vi "STFT by Indices.vi"(0 "scaled signal [EU]":dbl[](array[numeric]) format="%.2f", 1 "indices":i32[](array[numeric]), 2 "FFT block size":i32=1024, 5 "sampling frequency [Hz]":dbl=10000.0 format="%.2f", 7 "frequency weighting":T3(ring), 9 "window":T2 items=["Rectangle"=0, "Hanning"=1, "Hamming"=2, "Blackman-Harris"=3, "Exact Blackman"=4, "Blackman"=5, "Flat Top"=6, "4 Term B-Harris "=7, "7 Term B-Harris"=8, "Low Sidelobe"=9, "Blackman Nuttall"=11, "Triangle"=30, "Bartlett-Hanning"=31, "Bohman"=32, "Parzen"=33, "Welch"=34, "Kaiser"=60, "Dolph-Chebyshev"=61, "Gaussian"=62], 11 "channel info":T1={"sensor sensitivity [mV/EU]"=1000.0, "engineering units"=enum."V", "dB reference [EU]"=1.0, "custom label"="EU", "weighting filter"=enum."Linear", "pregain [dB]"=0.0} {"dB reference [EU]" format="%.1e"; "pregain [dB]" format="%.2f"; "sensor sensitivity [mV/EU]" format="%.2f"}, 12 "dB On (T)":bool=TRUE) -> (4 "power spectrum [EU^2 rms]":dbl[][](array[numeric]) format="%.2f", 6 "unit label":string, 8 "f0 and delta f [Hz]":cluster{"f0":dbl, "delta f":dbl} {"delta f" format="%.2f"; "f0" format="%.2f"}, 15 "weighting conflict":bool)   [LabVIEW 2017]
uses:
  <vilib>/Analysis/4window.llb/windowTd.ctl
  <vilib>/Analysis/NI_AALPro.lvlib
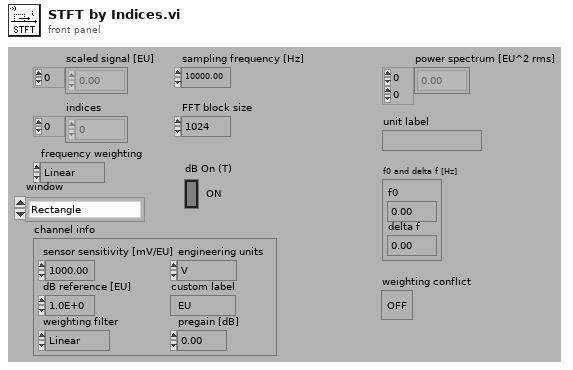
[diagram p1: front panel]
types:
  T1 = cluster{"sensor sensitivity [mV/EU]":dbl, "engineering units":enum16{"custom...", "V", "Pa", "g", "m/s^2", "m/s", "m", "in/s^2", "in/s", "in"}, "dB reference [EU]":dbl, "custom label":string, "weighting filter":enum16{"Linear", "A-weighting", "B-weighting", "C-weighting"}, "pregain [dB]":dbl}
  T2 = typedef "NI_AALPro.lvlib/windowTd.ctl" = u32
  T3 = enum16{"Linear", "A-weighting", "B-weighting", "C-weighting"}
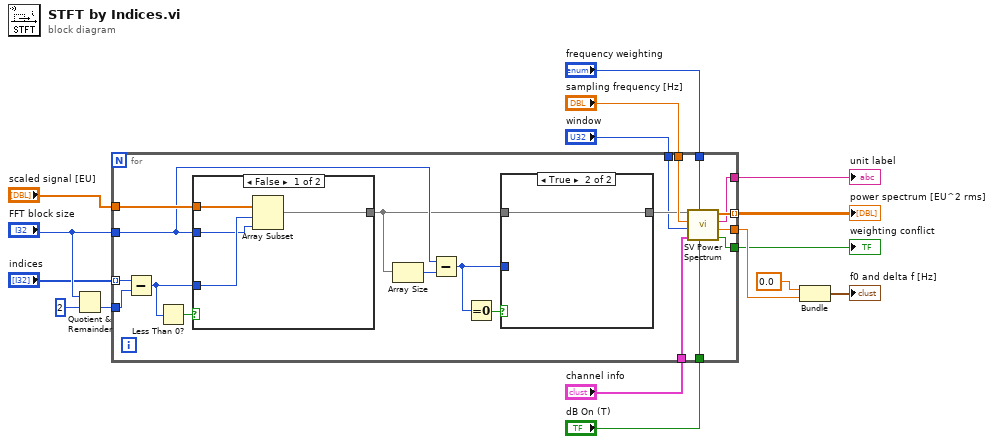
[diagram p0: block diagram]
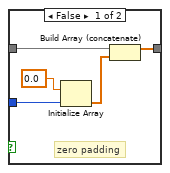
[diagram p2: hidden frame]
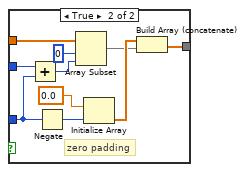
[diagram p3: hidden frame]
diagram:
  n1 = Quotient & Remainder(x="FFT block size", y=2) -> (floor(x/y)=w15:i32)  [unwired: 1 out]
  n2 = for {
    tunnel: w15 -> [w36]
    tunnel: "scaled signal [EU]" -> [w34]
    tunnel: "FFT block size" -> [w33]
    tunnel: "sampling frequency [Hz]" -> [w30]
    tunnel: [w29] -> w14 mode=indexing
    tunnel: [w27] -> w13
    tunnel: "frequency weighting" -> [w23]
    tunnel: "window" -> [w22]
    tunnel: "channel info" -> [w21]
    tunnel: "dB On (T)" -> [w20]
    tunnel: [w19] -> w5
    tunnel: [w18] -> w4
    tunnel: "indices" -> [w17] mode=indexing
    n3 = Subtract(x=w17, y=w36) -> (x-y=w35:i32)
    n4 = Less Than 0?(x=w35) -> (x < 0?=w28:bool)
    n5 = case shown="False" w28 {
      tunnel: w35 -> [w45 w52]
      tunnel: w34 -> [w46 w54]
      tunnel: w33 -> [w44 w50]
      tunnel: [w43 w47] -> w32
      frame False {
        n6 = Array Subset(array=w46, index=w45, length=w44) -> (w43:dbl[])
      }
      frame True {
        # "zero padding"
        n7 = Add(x=w50, y=w52) -> (x+y=w51:i32)
        n8 = Negate(x=w52) -> (-x=w56:i32)
        n9 = Array Subset(array=w54, index=0, length=w51) -> (w48:dbl[])
        n10 = Initialize Array(0.0, w56) -> (w49:dbl[])
        n11 = Build Array (concatenate)(w49, w48) -> (w47:dbl[])
      }
    }
    n12 = Array Size(array=w32) -> (size(s)=w26:i32)
    n13 = Subtract(x=w33, y=w26) -> (x-y=w31:i32)
    n14 = Equal To 0?(x=w31) -> (x = 0?=w25:bool)
    n15 = case shown="True" w25 {
      tunnel: [w37 w42] -> w24
      tunnel: w32 -> [w41 w42]
      tunnel: w31 -> [w39 _]
      frame False {
        # "zero padding"
        n16 = Initialize Array(0.0, w39) -> (w38:dbl[])
        n17 = Build Array (concatenate)(w41, w38) -> (w37:dbl[])
      }
      frame True {
      }
    }
    n18 = call <vilib>:"SV Power Spectrum.vi"("dB On (F)"=w20, "frequency weighting"=w23, "channel info"=w21, "window"=w22, "sampling frequency [Hz]"=w30, "scaled signal [EU]"=w24) -> ("weighting conflict"=w18:bool, "df [Hz]"=w27:dbl, "unit label"=w19:string, "power spectrum [EU^2 rms]"=w29:dbl[])  [unwired: 1 in, 1 out]
  }
  "power spectrum [EU^2 rms]" <- w14
  "unit label" <- w5
  "weighting conflict" <- w4
  n19 = Bundle(0.0, "df [Hz]"=w13) -> (→"f0 and delta f [Hz]":cluster{dbl, "df [Hz]":dbl})  [unwired: 1 in]
